vi "Save Data File.vi"(0 "File Type":T1, 5 "Data":dbl[][](array[numeric]) format="%0.2f", 7 "Number of Samples":i32, 9 "Open File Location?":bool, 11 "error in":errorcluster) -> (15 "error out":errorcluster)   [LabVIEW 2021]
uses:
  controls/File Type.ctl
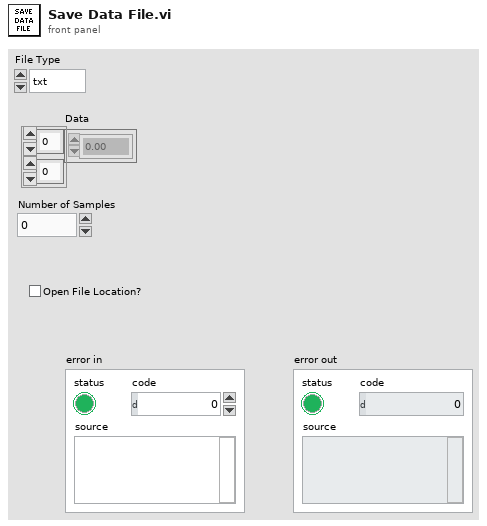
[diagram p1: front panel]
types:
  T1 = typedef "File Type.ctl" = enum16{"txt", "csv", "tdms"}
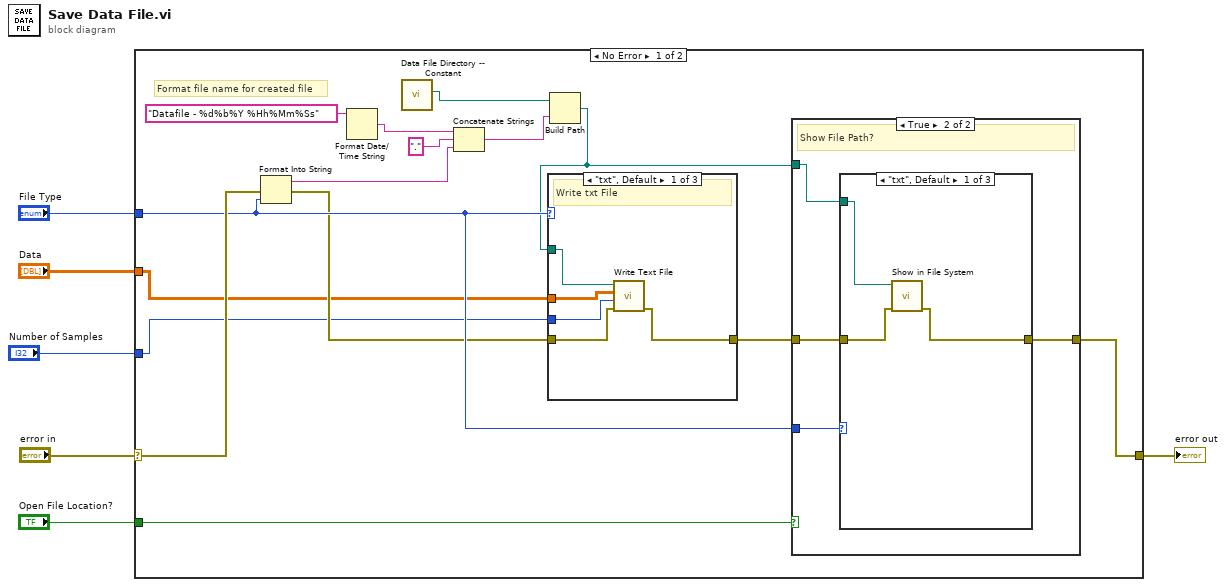
[diagram p0: block diagram]
diagram:
  n1 = case shown="No Error" "error in" {
    selector: "error in" -> [w21 w39]
    tunnel: [w16 w39] -> w5
    tunnel: "File Type" -> [w19 _]
    tunnel: "Data" -> [w8 _]
    tunnel: "Open File Location?" -> [w20 _]
    tunnel: "Number of Samples" -> [w7 _]
    frame No Error {
      # "Format file name for created file"
      n2 = Format Into String(error in=w21, w19) -> (resulting string=w13:string, error out=w18:errorcluster)  [unwired: 2 in]
      n3 = Format Date/Time String(time format string (%c)="Datafile - %d%b%Y %Hh%Mm%Ss") -> (date/time string=w15:string)  [unwired: 2 in]
      n4 = call "Data File Directory -- Constant.vi"() -> ("Data File Directory"=w11:path)  [unwired: 11 in]
      n5 = Concatenate Strings(w15, "." ("string"), w13) -> (w12:string)
      n6 = Build Path(base path=w11, name or relative path=w12) -> (appended path=w9:path)
      n7 = case shown="\"txt\", Default" w19 {
        tunnel: w18 -> [w36 w37 w38]
        tunnel: [w35 w37 w38] -> w17
        tunnel: w9 -> [w34 _ _]
        tunnel: w8 -> [w33 _ _]
        tunnel: w7 -> [w32 _ _]
        frame "txt", Default {
          # "Write txt File"
          n8 = call "Write Text File.vi"("error in"=w36, "Number of Samples"=w32, "Data In"=w33, "File Path"=w34) -> ("error out"=w35:errorcluster)  [unwired: 7 in]
        }
        frame "csv" {
          # "Write CSV File"
        }
        frame "tdms" {
          # "Write TDMS File"
        }
      }
      n9 = case shown="True" w20 {
        tunnel: w19 -> [_ w26]
        tunnel: w17 -> [w22 w25]
        tunnel: [w22 w24] -> w16
        tunnel: w9 -> [_ w23]
        frame False {
        }
        frame True {
          # "Show File Path?"
          n10 = case shown="\"txt\", Default" w26 {
            tunnel: w25 -> [w28 w30 w31]
            tunnel: [w27 w30 w31] -> w24
            tunnel: w23 -> [w29 _ _]
            frame "txt", Default {
              n11 = call <vilib>:"Show in File System.vi"("error in (no error)"=w28, "file or directory path"=w29) -> ("error out"=w27:errorcluster)  [unwired: 9 in]
            }
            frame "csv" {
            }
            frame "tdms" {
            }
          }
        }
      }
    }
    frame Error {
    }
  }
  "error out" <- w5
